vi "Send UnregisterAppenderMsg.vi"(8 "error in (no error)":errorcluster, 10 "id":string, 11 "Enqueuer in":refnum<class "Message Enqueuer.lvclass">) -> (0 "error out":errorcluster, 3 "Enqueuer out":refnum<class "Message Enqueuer.lvclass">)   [LabVIEW 2026, in "Lumberjack.lvlib" / "UnregisterAppenderMsg.lvclass"]
uses:
  UnregisterAppenderMsg.lvclass
  <vilib>/ActorFramework/Message Enqueuer/Message Enqueuer.lvclass
  UnregisterAppenderMsg.lvclass/UnregisterAppenderMsg.ctl
  <vilib>/ActorFramework/Message Enqueuer/Message Enqueuer.lvclass/Message Enqueuer.ctl
  <vilib>/ActorFramework/Message Priority Queue/Priority Enqueue.vi
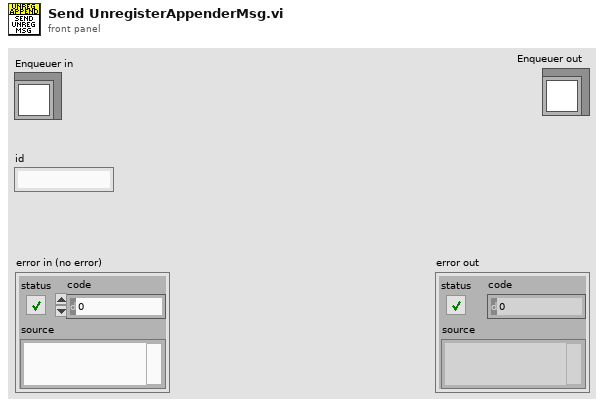
[diagram p1: front panel]
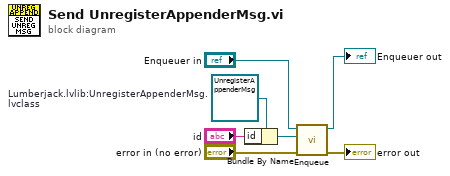
[diagram p0: block diagram]
diagram:
  w3 = refnum<class "UnregisterAppenderMsg.lvclass"> refnum  # Lumberjack.lvlib:UnregisterAppenderMsg.lvclass
  n1 = Bundle By Name(cluster=w3, "id"="id") -> (w1:refnum<class "UnregisterAppenderMsg.lvclass">)
  n2 = call <vilib>:"Enqueue.vi"("error in (no error)"="error in (no error)", "Message"=w1, "Message Enqueuer in"="Enqueuer in") -> ("error out"=→"error out":errorcluster, "Message Enqueuer out"=→"Enqueuer out":refnum<class "Message Enqueuer.lvclass">)  [unwired: 7 in]
